vi "Counter-Read_table.vi"(8 "Error In":errorcluster, 11 "task in":refnum<k21>) -> (0 "error out":errorcluster, 2 "time tags":u32[](array[numeric]))   [LabVIEW 2014]
uses:
  <vilib>/Utility/error.llb/DialogType.ctl
  <vilib>/DAQmx/read.llb/DAQmx Read (Counter 1D U32 1Chan NSamp).vi
  <vilib>/DAQmx/miscellaneous.llb/DAQmx Fill In Error Info.vi
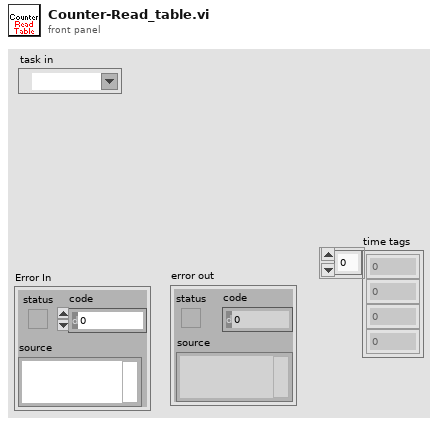
[diagram p1: front panel]
types:
  T1 = typedef "DialogType.ctl" = u16
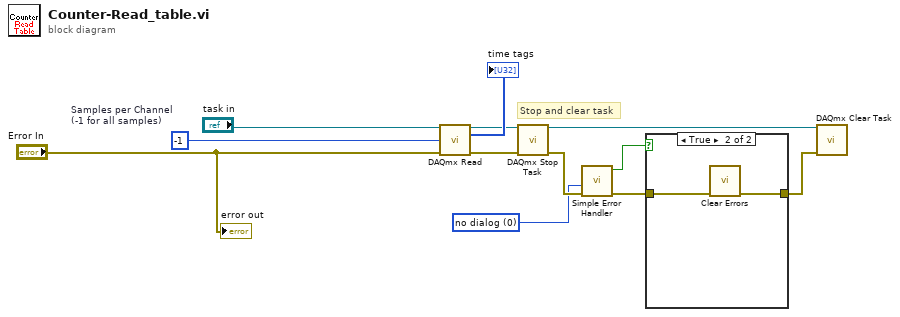
[diagram p0: block diagram]
diagram:
  w4 = T1 0 items=["no dialog", "OK message", "continue or stop message", "OK message + warnings", "continue/stop + warnings"] ("type of dialog (OK msg:1)")
  w11 = -1  # Samples per Channel  (-1 for all samples)
  # "Stop and clear task"
  n1 = call-poly <vilib>:"DAQmx Read.vi"("task/channels in"="task in", "number of samples per channel"=w11, "error in"="Error In") -> ("task out"=w7:refnum<k21>, "data"=→"time tags":u32[], "error out"=w6:errorcluster)  [unwired: 10 in]
  n2 = call <vilib>:"DAQmx Stop Task.vi"("task/channels in"=w7, "error in"=w6) -> ("task out"=w12:refnum<k21>, "error out"=w5:errorcluster)  [unwired: 12 in]
  n3 = call <vilib>:"Simple Error Handler.vi"("type of dialog (OK msg:1)"=w4, "error in (no error)"=w5) -> ("error?"=w3:bool, "error out"=w2:errorcluster)  [unwired: 3 in, 3 out]
  n4 = case shown="True" w3 {
    tunnel: w2 -> [w13 w15]
    tunnel: [w13 w14] -> w1
    frame False {
    }
    frame True {
      n5 = call <vilib>:"Clear Errors.vi"("error in (no error)"=w15) -> ("error out"=w14:errorcluster)  [unwired: 5 in, 1 out]
    }
  }
  n6 = call <vilib>:"DAQmx Clear Task.vi"("task in"=w12, "error in"=w1) -> ()  [unwired: 13 in, 1 out]
  "error out" <- "Error In"
